vi "Load System Config File.vi"(8 "error in (no error)":errorcluster, 11 "System Config in":T1) -> (0 "error out":errorcluster, 3 "System Config out":T1)   [LabVIEW 2026]
uses:
  controls/UI/System Config.ctl
  <vilib>/Utility/config.llb/Read Key (String).vi
  <vilib>/Utility/config.llb/Read Key (Path).vi
  <vilib>/Utility/config.llb/NI_LVConfig.lvlib
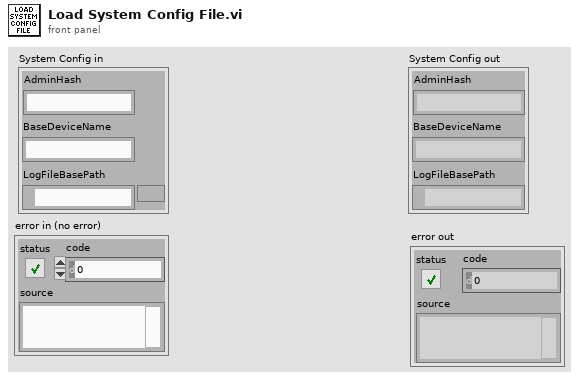
[diagram p1: front panel]
types:
  T1 = typedef "System Config.ctl" = cluster{"AdminHash":string, "BaseDeviceName":string, "LogFileBasePath ":path}
  T2 = typedef "NI_LVConfig.lvlib/Config Data RefNum.ctl" = refnum<k1>
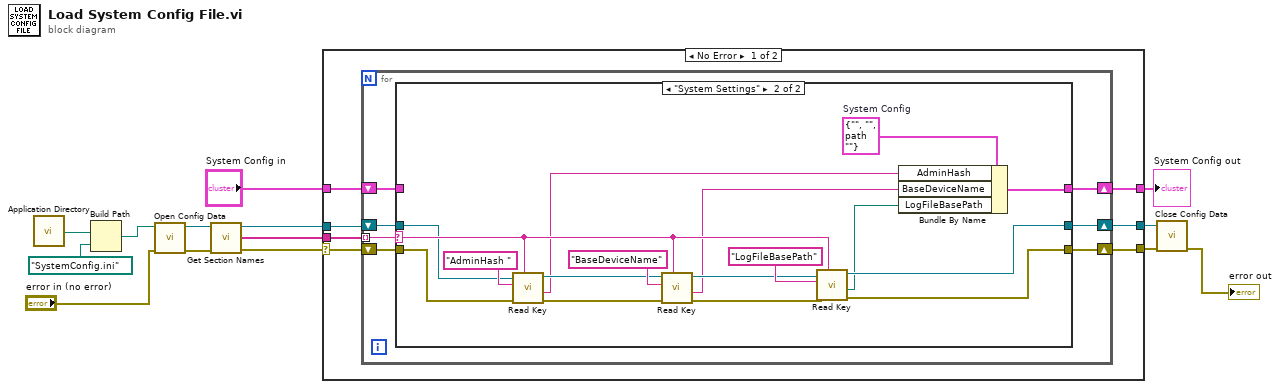
[diagram p0: block diagram]
diagram:
  n1 = call <vilib>:"Application Directory.vi"() -> ("Application Directory"=w13:path)
  n2 = Build Path(base path=w13, name or relative path=path "SystemConfig.ini" ("config file path")) -> (appended path=w12:path)
  n3 = call <vilib>:"Open Config Data.vi"("error in (no error)"="error in (no error)", "configuration file path"=w12) -> ("error out"=w10:errorcluster, "refnum"=w8:T2)  [unwired: 7 in, 1 out]
  n4 = call <vilib>:"Get Section Names.vi"("error in (no error)"=w10, "refnum"=w8) -> ("error out"=w9:errorcluster, "section names"=w7:string[], "refnum out"=w6:T2)  [unwired: 7 in]
  n5 = case shown="No Error" w9 {
    selector: w9 -> [w20 w51]
    tunnel: [w19 w51] -> w5
    tunnel: w7 -> [w21 _]
    tunnel: w6 -> [w17 w50]
    tunnel: [w18 w50] -> w3
    tunnel: [w16 w49] -> w2
    tunnel: "System Config in" -> [w15 w49]
    frame No Error {
      n6 = for {
        tunnel: w21 -> [w28] mode=indexing
        shift-right: [w27] -> w19
        shift-left: w20 -> [w24]
        shift-right: [w26] -> w18
        shift-left: w17 -> [w25]
        shift-right: [w23] -> w16
        shift-left: w15 -> [w22]
        n7 = case shown="\"System Settings\"" w28 {
          selector: w28 -> [_ w42]
          tunnel: [w31 w44] -> w27
          tunnel: [w30 w39] -> w26
          tunnel: w25 -> [w30 w38]
          tunnel: w24 -> [w31 w37]
          tunnel: [w29 w32] -> w23
          tunnel: w22 -> [w29 _]
          frame Default {
          }
          frame "System Settings" {
            w36 = T1 {"AdminHash"="", "BaseDeviceName"="", "LogFileBasePath "=path ""}  # System Config
            n8 = call-poly <vilib>:"Read Key.vi"("section"=w42, "error in (no error)"=w37, "key"="AdminHash ", "refnum"=w38) -> ("error out"=w46:errorcluster, "value"=w35:string, "refnum out"=w41:T2)  [unwired: 4 in, 1 out]
            n9 = call-poly <vilib>:"Read Key.vi"("section"=w42, "error in (no error)"=w46, "key"="BaseDeviceName", "refnum"=w41) -> ("error out"=w45:errorcluster, "value"=w34:string, "refnum out"=w40:T2)  [unwired: 4 in, 1 out]
            n10 = call-poly <vilib>:"Read Key.vi"("section"=w42, "error in (no error)"=w45, "key"="LogFileBasePath", "refnum"=w40) -> ("error out"=w44:errorcluster, "value"=w33:path, "refnum out"=w39:T2)  [unwired: 4 in, 1 out]
            n11 = Bundle By Name(cluster=w36, "AdminHash"=w35, "BaseDeviceName"=w34, "LogFileBasePath"=w33) -> (w32:T1)
          }
        }
      }
    }
    frame Error {
    }
  }
  "System Config out" <- w2
  n12 = call <vilib>:"Close Config Data.vi"("error in (no error)"=w5, "refnum"=w3) -> ("error out"=→"error out":errorcluster)  [unwired: 8 in, 1 out]
